vi "Plot Vectors.vi"(0 "picture in":picture, 5 "vectors":T1[](array[typedef]), 12 "pixy resolution":cluster{"width":u16, "height":u16}={"width"=79, "height"=52}, 13 "image resolution":cluster{"width":u16, "height":u16}={"width"=316, "height"=208}) -> (4 "picture out":picture)   [LabVIEW 2018, in "Pixy2.lvlib"]
uses:
  Pixy2.lvlib
  Types/Vector.ctl
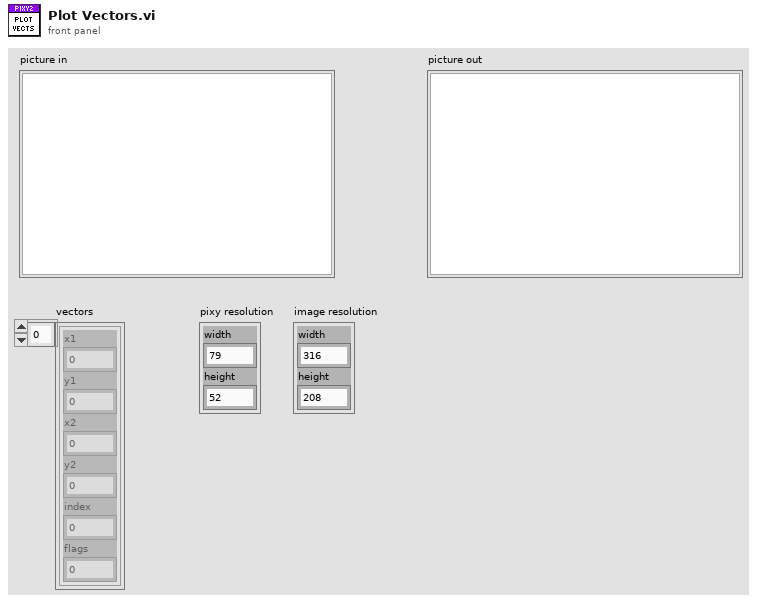
[diagram p1: front panel]
types:
  T1 = typedef "Pixy2.lvlib/Vector.ctl" = cluster{"x1":u8, "y1":u8, "x2":u8, "y2":u8, "index":u8, "flags":u8}
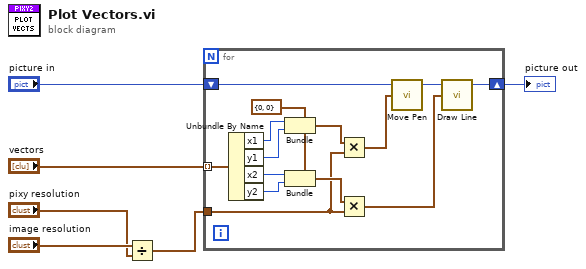
[diagram p0: block diagram]
diagram:
  n1 = Divide(x="image resolution", y="pixy resolution") -> (x/y=w1:cluster{"width":dbl, "height":dbl})
  n2 = for {
    shift-right: [w18] -> w5
    shift-left: "picture in" -> [w20]
    tunnel: "vectors" -> [w17] mode=indexing
    tunnel: w1 -> [w7]
    w12 = cluster{"x":i16, "y":i16} {"x"=0, "y"=0} ("new position")
    n3 = Unbundle By Name(w17) -> ("x1"=w16:u8, "y1"=w15:u8, "x2"=w14:u8, "y2"=w13:u8)
    n4 = Bundle(cluster=w12, "x"=w16, "y"=w15) -> (w9:cluster{"x":i16, "y":i16})
    n5 = Bundle(cluster=w12, "x"=w14, "y"=w13) -> (w11:cluster{"x":i16, "y":i16})
    n6 = Multiply(x=w9, y=w7) -> (x*y=w8:cluster{dbl, dbl})
    n7 = Multiply(x=w11, y=w7) -> (x*y=w10:cluster{dbl, dbl})
    n8 = call <vilib>:"Move Pen.vi"("new position"=w8, "picture"=w20) -> ("new picture"=w19:picture)  [unwired: 3 in]
    n9 = call <vilib>:"Draw Line.vi"("picture"=w19, "end point"=w10) -> ("new picture"=w18:picture)  [unwired: 7 in]
  }
  "picture out" <- w5
